vi "Functional Global - Control Configurations.vi"(7 "Functional Global Operation (Read)":T2=enum."Read", 11 "Control Configurations in":T1[](array[typedef])) -> (3 "Control Configurations out":T1[](array[typedef]))   [LabVIEW 2014]
uses:
  controls/Functional Global Operation.ctl
  controls/Control Configuration.ctl
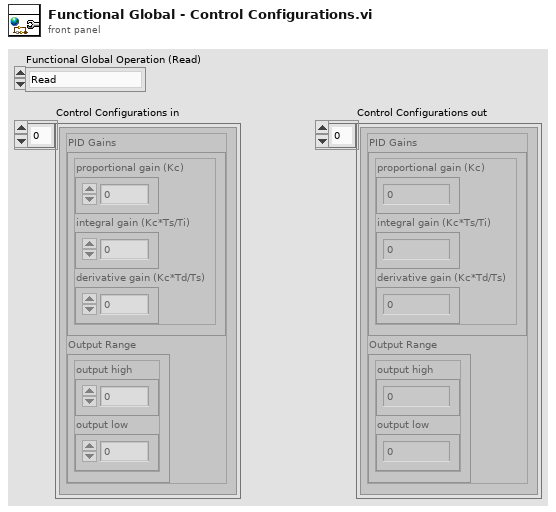
[diagram p1: front panel]
types:
  T1 = typedef "Control Configuration.ctl" = cluster{"PID Gains":cluster{"proportional gain (Kc)":dbl, "integral gain (Kc*Ts/Ti)":dbl, "derivative gain (Kc*Td/Ts)":dbl}, "Output Range":cluster{"output high":dbl, "output low":dbl}}
  T2 = typedef "Functional Global Operation.ctl" = enum16{"Initialize", "Read", "Write"}
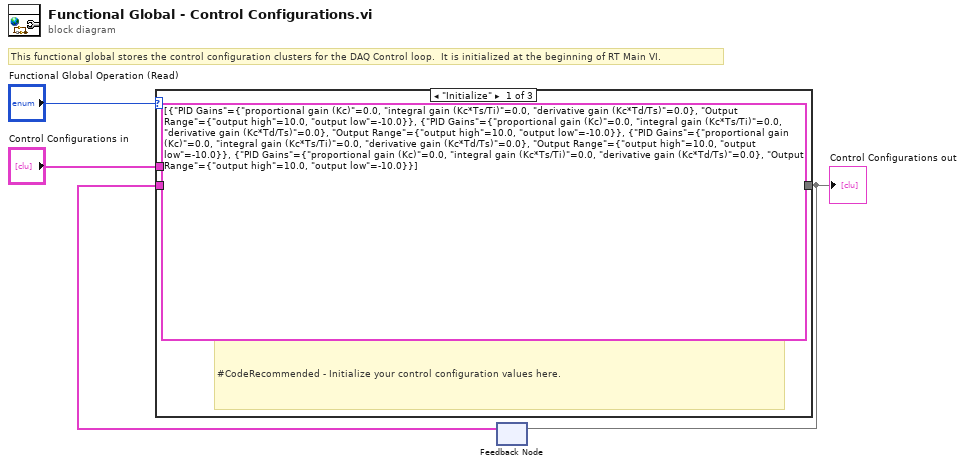
[diagram p0: block diagram]
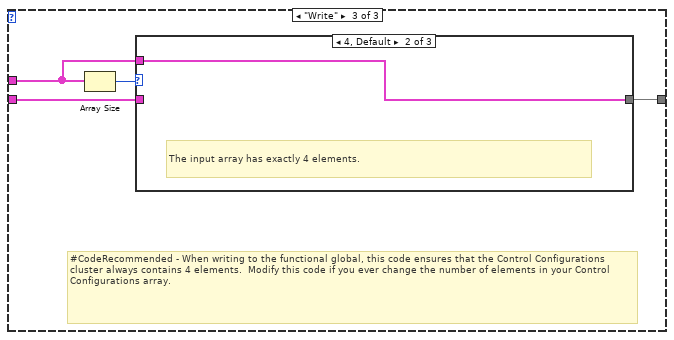
[diagram p3: hidden frame]
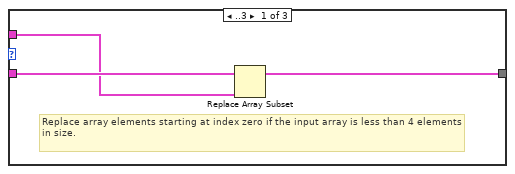
[diagram p4: hidden frame]
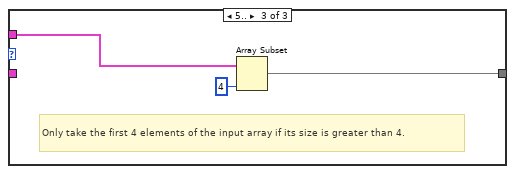
[diagram p5: hidden frame]
diagram:
  # "This functional global stores the control configuration clusters for the DAQ Control loop.  It is initialized at the beginning of RT Main VI."
  n1 = feedback #1() -> (w1:T1[])  [unwired: 1 in]
  n2 = case shown="\"Initialize\"" "Functional Global Operation (Read)" {
    tunnel: "Control Configurations in" -> [_ _ w8]
    tunnel: [T1[] [{"PID Gains"={"proportional gain (Kc)"=0.0, "integral gain (Kc*Ts/Ti)"=0.0, "derivative gain (Kc*Td/Ts)"=0.0}, "Output Range"={"output high"=10.0, "output low"=-10.0}}, {"PID Gains"={"proportional gain (Kc)"=0.0, "integral gain (Kc*Ts/Ti)"=0.0, "derivative gain (Kc*Td/Ts)"=0.0}, "Output Range"={"output high"=10.0, "output low"=-10.0}}, {"PID Gains"={"proportional gain (Kc)"=0.0, "integral gain (Kc*Ts/Ti)"=0.0, "derivative gain (Kc*Td/Ts)"=0.0}, "Output Range"={"output high"=10.0, "output low"=-10.0}}, {"PID Gains"={"proportional gain (Kc)"=0.0, "integral gain (Kc*Ts/Ti)"=0.0, "derivative gain (Kc*Td/Ts)"=0.0}, "Output Range"={"output high"=10.0, "output low"=-10.0}}] ("Control Configurations in") w6 w7] -> w2
    tunnel: w1 -> [_ w6 w9]
    frame "Initialize" {
      # "#CodeRecommended - Initialize your control configuration values here."
    }
    frame "Read", Default {
    }
    frame "Write" {
      # "#CodeRecommended - When writing to the functional global, this code ensures that the Control Configurations cluster always contains 4 elements.  Modify this code if you ever change the number of elements in your Control Configurations array."
      n3 = Array Size(array=w8) -> (size(s)=w10:i32)
      n4 = case shown="4, Default" w10 {
        tunnel: w9 -> [w13 _ _]
        tunnel: w8 -> [w12 w14 w17]
        tunnel: [w11 w14 w15] -> w7
        frame ..3 {
          # "Replace array elements starting at index zero if the input array is less than 4 elements in size."
          n5 = Replace Array Subset(array=w13, new element=w12) -> (w11:T1[])  [unwired: 1 in]
        }
        frame 4, Default {
          # "The input array has exactly 4 elements."
        }
        frame 5.. {
          # "Only take the first 4 elements of the input array if its size is greater than 4."
          n6 = Array Subset(array=w17, length=4) -> (w15:T1[])  [unwired: 1 in]
        }
      }
    }
  }
  "Control Configurations out" <- w2
  n7 = feedback-in #1(w2) -> ()
